vi "subAdd2TierProjectItems.vi"(8 "error in (no error)":errorcluster, 9 "ProjectItems":refnum<class "ProjectItem.lvclass">[](array[class]), 10 "Owning project":path, 11 "SolutionBuilder in":refnum<class "SolutionBuilder.lvclass">) -> (0 "error out":errorcluster, 3 "SolutionBuilder out":refnum<class "SolutionBuilder.lvclass">)   [LabVIEW 2020, in "SolutionBuilder.lvlib" / "SolutionBuilder.lvclass"]
uses:
  SolutionBuilder.lvclass
  <vilib>/Utility/miscctls.llb/LVMapReplaceAction.ctl
  ProjectItem/ProjectItem.lvclass
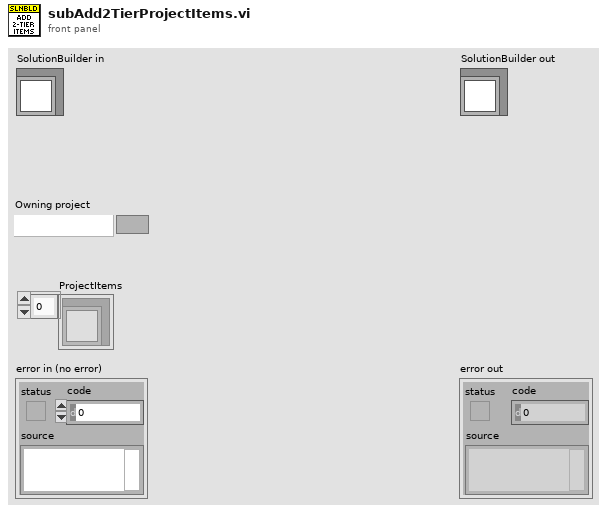
[diagram p1: front panel]
types:
  T1 = typedef "LVMapReplaceAction.ctl" = enum32{"Modify Entry only if found", "Add or Modify Entry", "Delete Entry"}
  T2 = typedef "SolutionBuilder.lvlib/SolutionBuilder.lvclass/ProjectItemMap.ctl" = map{path, refnum<class "ProjectItem.lvclass">[]}
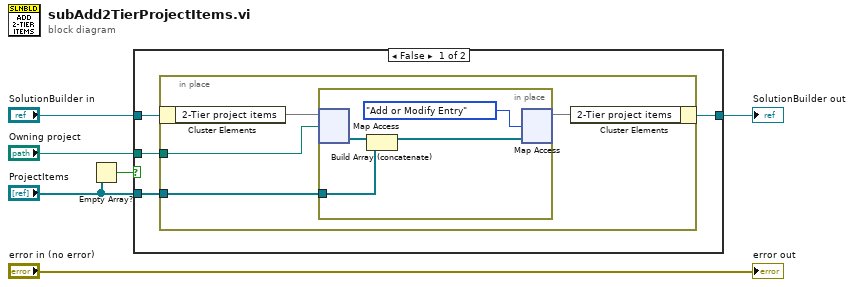
[diagram p0: block diagram]
diagram:
  n1 = Empty Array?(array="ProjectItems") -> (empty?=w1:bool)
  n2 = case shown="False" w1 {
    tunnel: "SolutionBuilder in" -> [w10 w19]
    tunnel: "Owning project" -> [w9 _]
    tunnel: "ProjectItems" -> [w8 _]
    tunnel: [w7 w19] -> w3
    frame False {
      n3 = in-place {
        in-place-border: w9 -> [w12]
        in-place-border: w8 -> [w14]
        n4 = in-place-cluster #1(w10) -> ("2-Tier project items"=w13:T2)
        n5 = in-place {
          in-place-border: w14 -> [w17]
          n6 = in-place-map #2(w13, w12) -> (w18:refnum<class "ProjectItem.lvclass">[])  [unwired: 1 in, 1 out]
          n7 = Build Array (concatenate)(w18, w17) -> (w16:refnum<class "ProjectItem.lvclass">[])
          n8 = in-place-map #2(w16, LVMapReplaceAction."Add or Modify Entry" ("action")) -> (w11:T2)  [unwired: 2 out]
        }
        n9 = in-place-cluster #1("2-Tier project items"=w11) -> (w7:refnum<class "SolutionBuilder.lvclass">)
      }
    }
    frame True {
    }
  }
  "SolutionBuilder out" <- w3
  "error out" <- "error in (no error)"
